vi "溶解氧电极校准.vi"() -> ()   [LabVIEW 2016, in "斯坦道多参数.lvlib"]
uses:
  <vilib>/Utility/miscctls.llb/LVPointTypeDef.ctl
  <vilib>/Analysis/NI_AALBase.lvlib
panel:
  out "第二点校准值":dbl
  out "第一点校准值":dbl
  out "最小值":sgl format="%#.2f"
  out "最大值":sgl format="%#.2f"
  in  "校准模式":enum16{"两点校准", "单点校准"}(ring)=enum."单点校准"
  in  "校准停止":bool
  in  "校准启动":bool
  out "波形图表":sgl(graph) caption="历史曲线"
  out "变异系数":dbl format="%#.6f"
  out "standard deviation":dbl caption="标准差" format="%#.2f"
  out "mean":dbl caption="均值" format="%#.2f"
  out "测量读值":dbl
  out "偏移值补偿":dbl
  out "饱和度值":dbl
  out "提示":string
  out "气压补偿值":dbl
  out "盐度补偿值":dbl
  out "电极斜率":dbl
  out "电极零点":dbl
  # "溶解氧电极设定"
  # "%"
  # "%"
  # "%"
  # "mg/L"
  # "ppt"
  # "hPa"
  # "mg/L"
  # "请选择校准模式:"
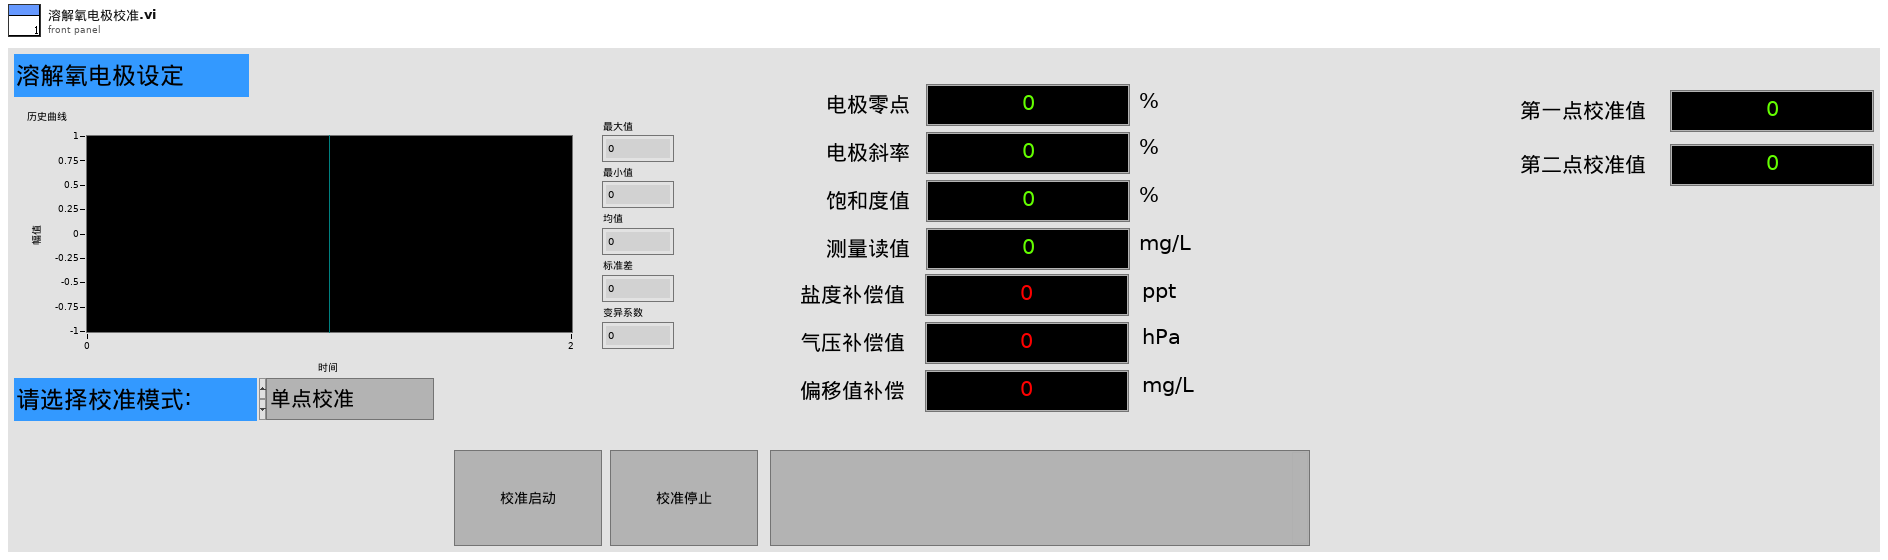
[diagram p1: front panel]
types:
  T1 = typedef "斯坦道多参数.lvlib/校准步骤.ctl" = enum16{"待机", "放置第一点标液", "第一点校准启动", "第一点校准写入", "第一点校准失败", "放置第二点标液", "第二点校准启动", "第二点校准写入", "第二点校准失败", "校准结果写入", "校准结束"}
  T2 = typedef "LVPointTypeDef.ctl" = cluster{"Horizontal":i16, "Vertical":i16}
  T3 = cluster{"电极状态标志":u16, "电极型号标志":u16, "溶解氧测量值":sgl, "温度测量值":sgl, "溶解氧饱和度值":sgl, "盐度补偿值":sgl, "大气压补偿值":sgl, "溶解氧偏移修正值":sgl, "温度偏移修正值":sgl, "手动温度补偿值":sgl, "溶解氧电极零点":sgl, "溶解氧电极斜率":sgl, "第1点标准值记录":sgl, "第1点信号值记录":sgl, "第1点温度值记录":sgl, "第2点标准值记录":sgl, "第2点信号值记录":sgl, "第2点温度值记录":sgl, "命令滤波设定":u16, "温度模式":enum16{"ATC", "MTC"}, "生产批次":u16, "电极序号":u16, "串口地址":u16, "串口波特率":enum16{"9600", "19200", "115200"}, "串口校验位":enum16{"NONE", "ODD", "EVEN"}, "串口停止位":enum16{"1bit", "2bit"}, "第一点标准值":sgl, "第二点标准值":sgl}
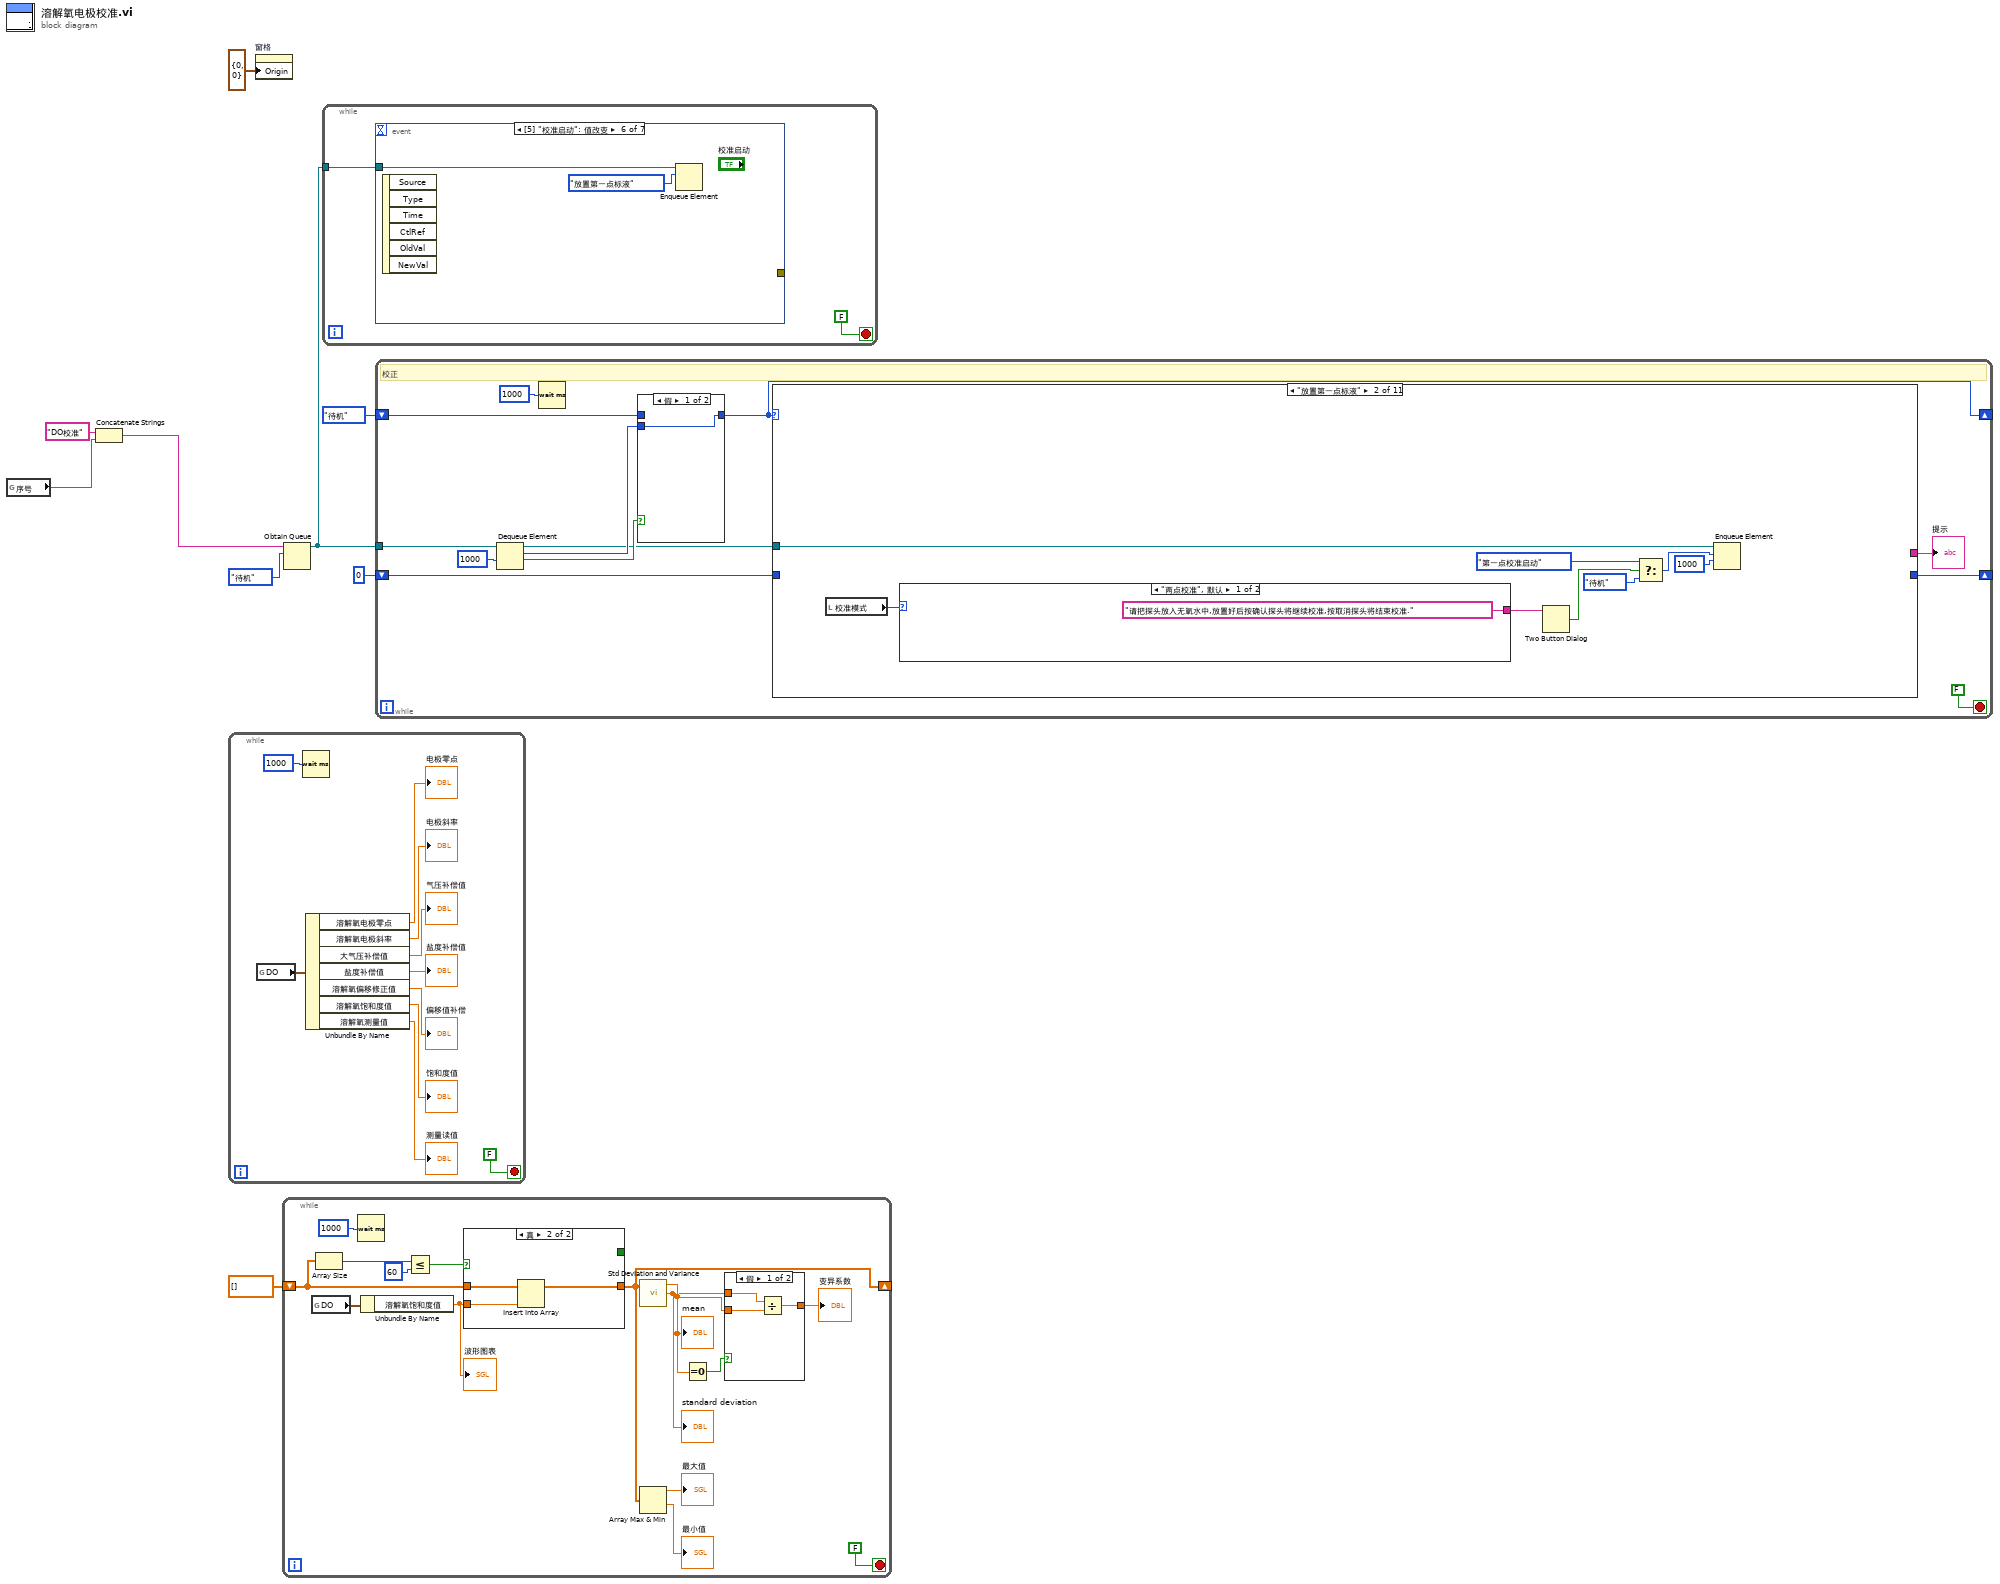
[diagram p0: block diagram]
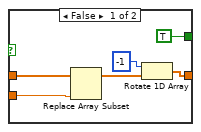
[diagram p3: hidden frame]
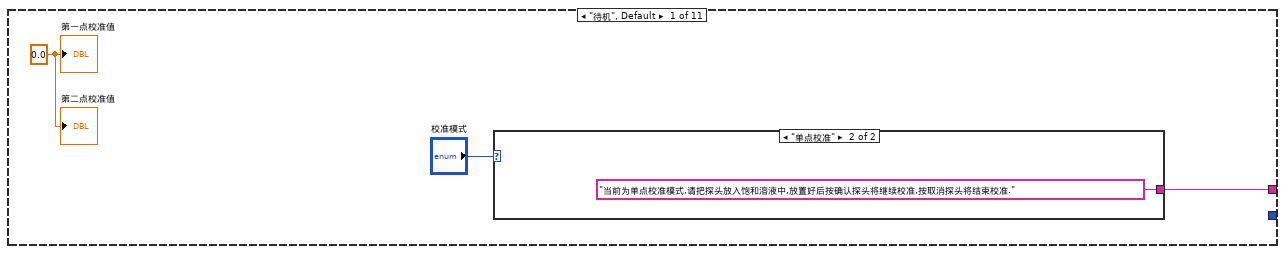
[diagram p5: hidden frame]
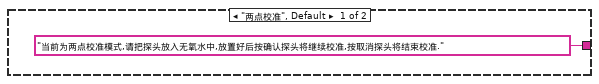
[diagram p6: hidden frame]
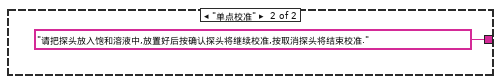
[diagram p7: hidden frame]
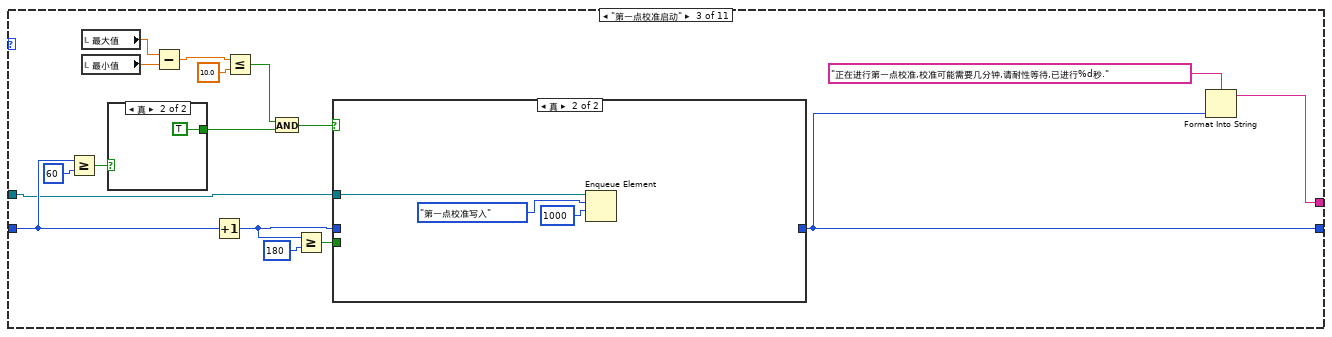
[diagram p8: hidden frame]
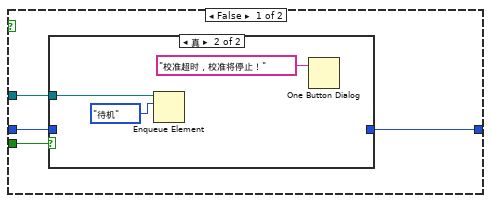
[diagram p9: hidden frame]
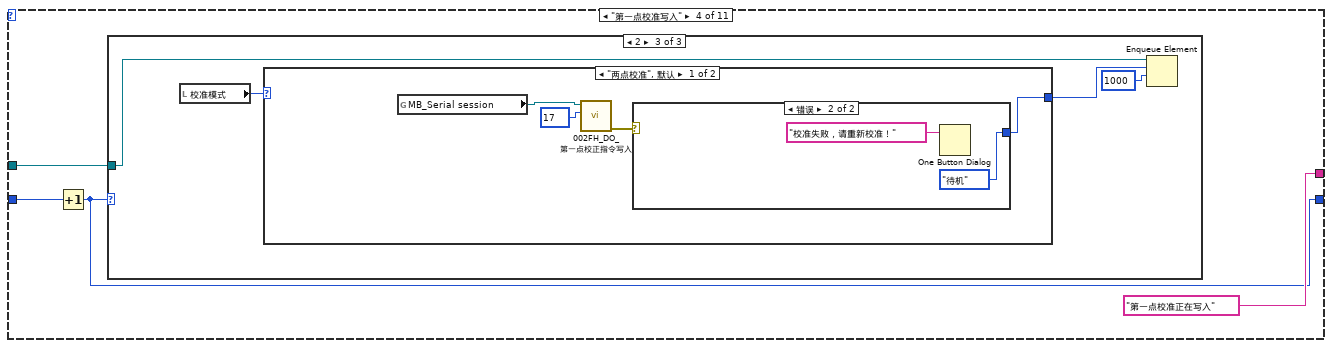
[diagram p12: hidden frame]
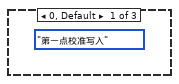
[diagram p13: hidden frame]
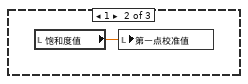
[diagram p14: hidden frame]
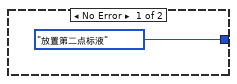
[diagram p15: hidden frame]
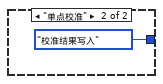
[diagram p16: hidden frame]
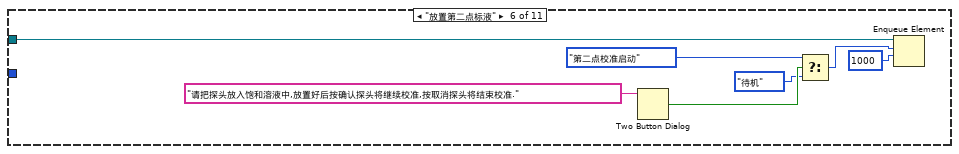
[diagram p18: hidden frame]
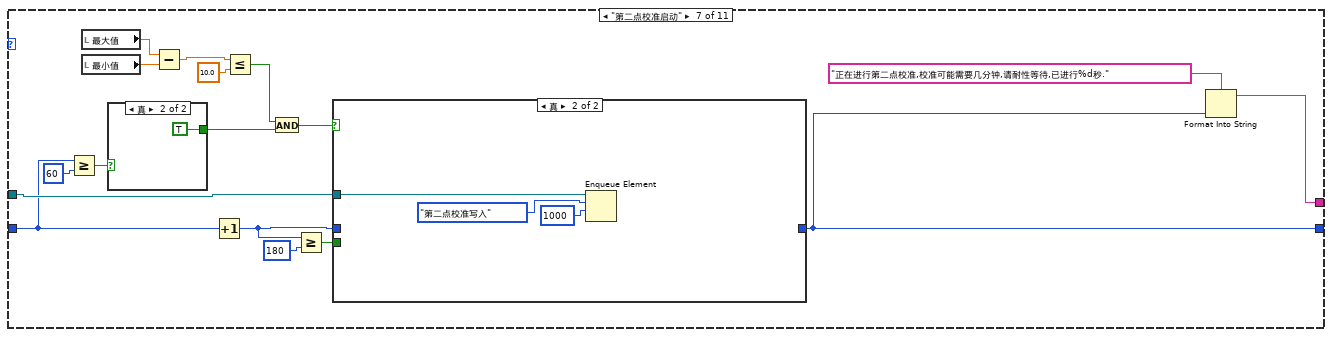
[diagram p19: hidden frame]
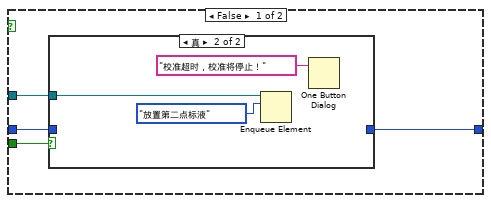
[diagram p20: hidden frame]
diagram:
  n1 = global read "多参数全局变量.vi" "序号"() -> (w1:string)
  n2 = Concatenate Strings("DO校准" ("名称（未命名）"), w1) -> (w2:string)
  n3 = while {
    stop <- FALSE stop-if-true
    n4 = global read "国弘过程全局变量.vi" "DO"() -> (w17:T3)
    n5 = Wait (ms)(milliseconds to wait=u32 1000 ("等待时间（毫秒）")) -> ()  [unwired: 1 out]
    n6 = Unbundle By Name(w17) -> ("溶解氧电极零点"=→"电极零点":sgl, "溶解氧电极斜率"=→"电极斜率":sgl, "大气压补偿值"=→"气压补偿值":sgl, "盐度补偿值"=→"盐度补偿值":sgl, "溶解氧偏移修正值"=→"偏移值补偿":sgl, "溶解氧饱和度值"=→"饱和度值":sgl, "溶解氧测量值"=→"测量读值":sgl)
  }
  n7 = property on="窗格" class="Pane"("Origin"=T2 {"Horizontal"=0, "Vertical"=0} ("原点")) -> ()  [unwired: 2 in, 2 out]
  n8 = while {
    shift-right: [w23] -> _
    shift-left: sgl[] [] -> [w30]
    stop <- FALSE stop-if-true
    n9 = global read "国弘过程全局变量.vi" "DO"() -> (w26:T3)
    n10 = Array Size(array=w30) -> (size(s)=w32:i32)
    n11 = Wait (ms)(milliseconds to wait=u32 1000 ("等待时间（毫秒）")) -> ()  [unwired: 1 out]
    n12 = Unbundle By Name(w26) -> ("溶解氧饱和度值"=w20:sgl)
    "波形图表" <- w20
    n13 = Less Or Equal?(x=w32, y=60) -> (x <= y?=w31:bool)
    n14 = case shown="真" w31 {
      tunnel: w30 -> [w43 w46]
      tunnel: w20 -> [w41 w45]
      tunnel: [w39 w44] -> w23
      tunnel: [TRUE _] -> _
      frame False {
        n15 = Replace Array Subset(array=w43, new element=w41) -> (w42:sgl[])  [unwired: 1 in]
        n16 = Rotate 1D Array(1:w42, 2:-1 ("n")) -> (0:w39:sgl[])
      }
      frame True {
        n17 = Insert Into Array(array=w46, new element=w45) -> (w44:sgl[])  [unwired: 1 in]
      }
    }
    n18 = call <vilib>:"Std Deviation and Variance.vi"("X"=w23) -> ("mean"=w25:dbl, "standard deviation"=w24:dbl)  [unwired: 1 in, 1 out]
    "mean" <- w25
    "standard deviation" <- w24
    n19 = Array Max & Min(array=w23) -> (max value=→"最大值":sgl, min value=→"最小值":sgl)  [unwired: 2 out]
    n20 = Equal To 0?(x=w25) -> (x = 0?=w29:bool)
    n21 = case shown="假" w29 {
      tunnel: w24 -> [w37 _]
      tunnel: [w36 _] -> w28
      tunnel: w25 -> [w35 _]
      frame False {
        n22 = Divide(x=w37, y=w35) -> (x/y=w36:dbl)
      }
      frame True {
      }
    }
    "变异系数" <- w28
  }
  n23 = Obtain Queue(name (unnamed)=w2, element data type=校准步骤."待机" ("枚举")) -> (queue out=w3:refnum<queue>)  [unwired: 3 in, 2 out]
  n24 = while {
    tunnel: w3 -> [w47]
    stop <- FALSE stop-if-true
    n25 = event shown="[5] \"校准启动\": 值改变" {
      selector: _ -> [_ _ _ _ _ _ _]
      dyn-events: _ -> [_ _ _ _ _ _ _]
      timeout: _ -> [_ _ _ _ _ _ _]
      tunnel: [_ _ w54 w57 w60 _ _] -> _
      tunnel: w47 -> [_ _ _ _ _ w62 w64]
      event Timeout {
        n26 = event-data() -> ()  [unwired: 1 in, 3 out]
      }
      event "盐度补偿值", "气压补偿值", "偏移值补偿": Mouse Down {
        n27 = event-data() -> ("CtlRef"=w50:refnum<vi>)  [unwired: 1 in, 7 out]
        n28 = property class="DigNum (严格)"(reference=w50) -> (reference out=w49:refnum<vi>, "Value"=w51:dbl)  [unwired: 1 in, 1 out]
        n29 = call "数字键盘.vi"("OldNumber"=w51) -> ("NewNumber"=w52:sgl)
        n30 = property class="DigNum (严格)"(reference=w49, "Val(Sgnl)"=w52) -> ()  [unwired: 1 in, 2 out]
      }
      event "盐度补偿值": Value Change {
        n31 = event-data() -> ("NewVal"=w55:dbl)  [unwired: 1 in, 5 out]
        n32 = global read "多参数全局变量.vi" "MB_Serial session"() -> (w53:refnum<class "MB_Master_Serial.lvclass">)
        n33 = call "0008H_DO_盐度补偿值写入.vi"("数值"=w55, "MB_Serial session in"=w53) -> ("error out"=w54:errorcluster)  [unwired: 8 in, 1 out]
      }
      event "气压补偿值": Value Change {
        n34 = event-data() -> ("NewVal"=w58:dbl)  [unwired: 1 in, 5 out]
        n35 = global read "多参数全局变量.vi" "MB_Serial session"() -> (w56:refnum<class "MB_Master_Serial.lvclass">)
        n36 = call "000AH_DO_大气压补偿值写入.vi"("数值"=w58, "MB_Serial session in"=w56) -> ("error out"=w57:errorcluster)  [unwired: 8 in, 1 out]
      }
      event "偏移值补偿": Value Change {
        n37 = event-data() -> ("NewVal"=w61:dbl)  [unwired: 1 in, 5 out]
        n38 = global read "多参数全局变量.vi" "MB_Serial session"() -> (w59:refnum<class "MB_Master_Serial.lvclass">)
        n39 = call "000CH_DO_DO偏移修正值写入.vi"("数值"=w61, "MB_Serial session in"=w59) -> ("error out"=w60:errorcluster)  [unwired: 8 in, 1 out]
      }
      event "校准启动": Value Change {
        n40 = event-data() -> ()  [unwired: 1 in, 6 out]
        n41 = Enqueue Element(queue=w62, element=校准步骤."放置第一点标液" ("元素")) -> ()  [unwired: 2 in, 3 out]
      }
      event "校准停止": Value Change {
        n42 = event-data() -> ()  [unwired: 1 in, 6 out]
        n43 = Flush Queue(queue=w64) -> (queue out=w65:refnum<queue>)  [unwired: 1 in, 2 out]
        n44 = Enqueue Element(queue=w65, element=校准步骤."待机" ("元素"), timeout in ms (-1)=1000 ("超时毫秒(-1)")) -> ()  [unwired: 1 in, 3 out]
      }
    }
  }
  n45 = while "While循环" {
    shift-right: [w69] -> _
    shift-left: 校准步骤."待机" ("枚举") -> [w70]
    shift-right: [w76] -> _
    shift-left: 0 -> [w77]
    tunnel: w3 -> [w71]
    stop <- FALSE stop-if-true
    # "校正"
    n46 = Dequeue Element(queue=w71, timeout in ms (-1)=1000 ("超时毫秒(-1)")) -> (queue out=w68:refnum<queue>, element=w72:T1, timed out?=w73:bool)  [unwired: 1 in, 1 out]
    n47 = Wait (ms)(milliseconds to wait=u32 1000 ("等待时间（毫秒）")) -> ()  [unwired: 1 out]
    n48 = case shown="假" w73 {
      tunnel: w72 -> [w80 _]
      tunnel: [w80 w81] -> w69
      tunnel: w70 -> [_ w81]
      frame False {
      }
      frame True {
      }
    }
    n49 = case shown="\"放置第一点标液\"" w69 {
      tunnel: [w84 _ w101 "第一点校准正在写入" ("提示") _ _ w151 "第二点校准正在写入" ("提示") _ w193 w221] -> w75
      tunnel: w77 -> [_ _ w105 w128 _ _ w153 w181 _ _ _]
      tunnel: [_ _ w104 w127 _ _ w152 w180 _ _ _] -> w76
      tunnel: w68 -> [_ w88 w103 w126 _ w143 w154 w179 _ w195 _]
      frame "待机", Default {
        w82 = 0.0 ("第一点校准值")
        n50 = case shown="\"单点校准\"" "校准模式" {
          tunnel: ["当前为两点校准模式,请把探头放入无氧水中,放置好后按确认探头将继续校准,按取消探头将结束校准." ("消息") "当前为单点校准模式,请把探头放入饱和溶液中,放置好后按确认探头将继续校准,按取消探头将结束校准." ("消息")] -> w84
          frame "两点校准", Default {
          }
          frame "单点校准" {
          }
        }
        "第一点校准值" <- w82
        "第二点校准值" <- w82
      }
      frame "放置第一点标液" {
        n51 = local read "校准模式"() -> (w87:enum16{"两点校准", "单点校准"})
        n52 = case shown="\"两点校准\", 默认" w87 {
          tunnel: ["请把探头放入无氧水中,放置好后按确认探头将继续校准,按取消探头将结束校准." ("消息") "请把探头放入饱和溶液中,放置好后按确认探头将继续校准,按取消探头将结束校准." ("消息")] -> w94
          frame "两点校准", Default {
          }
          frame "单点校准" {
          }
        }
        n53 = Two Button Dialog(message=w94) -> (T button?=w92:bool)  [unwired: 2 in]
        n54 = Select(t=校准步骤."第一点校准启动" ("元素"), s=w92, f=校准步骤."待机" ("元素")) -> (s? t:f=w89:T1)
        n55 = Enqueue Element(queue=w88, element=w89, timeout in ms (-1)=1000 ("超时毫秒(-1)")) -> ()  [unwired: 1 in, 3 out]
      }
      frame "第一点校准启动" {
        n56 = Greater Or Equal?(x=w105, y=60) -> (x >= y?=w112:bool)
        n57 = local read "最大值"() -> (w109:sgl)
        n58 = local read "最小值"() -> (w108:sgl)
        n59 = case shown="真" w112 {
          tunnel: [_ TRUE] -> w100
          frame False {
          }
          frame True {
          }
        }
        n60 = Subtract(x=w109, y=w108) -> (x-y=w110:sgl)
        n61 = Increment(x=w105) -> (x+1=w102:i32)
        n62 = Less Or Equal?(x=w110, y=10.0) -> (x <= y?=w99:bool)
        n63 = And(x=w99, y=w100) -> (x .and. y?=w98:bool)
        n64 = Greater Or Equal?(x=w102, y=180) -> (x >= y?=w106:bool)
        n65 = case shown="真" w98 {
          tunnel: w103 -> [w116 w124]
          tunnel: w106 -> [w117 _]
          tunnel: w102 -> [w115 _]
          tunnel: [w114 _] -> w104
          frame False {
            n66 = case shown="真" w117 {
              tunnel: w116 -> [_ w121]
              tunnel: w115 -> [w118 _]
              tunnel: [w118 _] -> w114
              frame False {
              }
              frame True {
                n67 = Enqueue Element(queue=w121, element=校准步骤."待机" ("元素")) -> ()  [unwired: 2 in, 3 out]
                n68 = One Button Dialog(message="校准超时，校准将停止！" ("消息")) -> ()  [unwired: 1 in, 1 out]
              }
            }
          }
          frame True {
            n69 = Enqueue Element(queue=w124, element=校准步骤."第一点校准写入" ("元素"), timeout in ms (-1)=1000 ("超时毫秒(-1)")) -> ()  [unwired: 1 in, 3 out]
          }
        }
        n70 = Format Into String(format string="正在进行第一点校准,校准可能需要几分钟,请耐性等待,已进行%d秒." ("格式字符串"), w104) -> (resulting string=w101:string)  [unwired: 2 in, 1 out]
      }
      frame "第一点校准写入" {
        n71 = Increment(x=w128) -> (x+1=w127:i32)
        n72 = case shown="2" w127 {
          tunnel: w126 -> [_ _ w132]
          frame 0, Default {
            (unwired) 校准步骤."第一点校准写入" ("枚举")
          }
          frame 1 {
            n73 = local read "饱和度值"() -> (w130:dbl)
            n74 = local write "第一点校准值"(w130) -> ()
          }
          frame 2 {
            n75 = local read "校准模式"() -> (w134:enum16{"两点校准", "单点校准"})
            n76 = case shown="\"两点校准\", 默认" w134 {
              tunnel: [w135 校准步骤."校准结果写入" ("枚举")] -> w131
              frame "两点校准", Default {
                n77 = global read "多参数全局变量.vi" "MB_Serial session"() -> (w136:refnum<class "MB_Master_Serial.lvclass">)
                n78 = call "002FH_DO_第一点校正指令写入.vi"("数值"=u16 17, "MB_Serial session in"=w136) -> ("error out"=w137:errorcluster)  [unwired: 8 in, 1 out]
                n79 = case shown="错误" w137 {
                  tunnel: [校准步骤."放置第二点标液" ("元素") 校准步骤."待机" ("元素")] -> w135
                  frame No Error {
                  }
                  frame Error {
                    n80 = One Button Dialog(message="校准失败，请重新校准！" ("消息")) -> ()  [unwired: 1 in, 1 out]
                  }
                }
              }
              frame "单点校准" {
              }
            }
            n81 = Enqueue Element(queue=w132, element=w131, timeout in ms (-1)=1000 ("超时毫秒(-1)")) -> ()  [unwired: 1 in, 3 out]
          }
        }
      }
      frame "第一点校准失败" {
      }
      frame "放置第二点标液" {
        n82 = Two Button Dialog(message="请把探头放入饱和溶液中,放置好后按确认探头将继续校准,按取消探头将结束校准." ("消息")) -> (T button?=w147:bool)  [unwired: 2 in]
        n83 = Select(t=校准步骤."第二点校准启动" ("元素"), s=w147, f=校准步骤."待机" ("元素")) -> (s? t:f=w144:T1)
        n84 = Enqueue Element(queue=w143, element=w144, timeout in ms (-1)=1000 ("超时毫秒(-1)")) -> ()  [unwired: 1 in, 3 out]
      }
      frame "第二点校准启动" {
        n85 = Greater Or Equal?(x=w153, y=60) -> (x >= y?=w165:bool)
        n86 = local read "最大值"() -> (w162:sgl)
        n87 = local read "最小值"() -> (w161:sgl)
        n88 = case shown="真" w165 {
          tunnel: [_ TRUE] -> w158
          frame False {
          }
          frame True {
          }
        }
        n89 = Subtract(x=w162, y=w161) -> (x-y=w163:sgl)
        n90 = Increment(x=w153) -> (x+1=w159:i32)
        n91 = Less Or Equal?(x=w163, y=10.0) -> (x <= y?=w157:bool)
        n92 = And(x=w157, y=w158) -> (x .and. y?=w156:bool)
        n93 = Greater Or Equal?(x=w159, y=180) -> (x >= y?=w160:bool)
        n94 = case shown="真" w156 {
          tunnel: w154 -> [w169 w177]
          tunnel: w160 -> [w170 _]
          tunnel: w159 -> [w168 _]
          tunnel: [w167 _] -> w152
          frame False {
            n95 = case shown="真" w170 {
              tunnel: w169 -> [_ w174]
              tunnel: w168 -> [w171 _]
              tunnel: [w171 _] -> w167
              frame False {
              }
              frame True {
                n96 = Enqueue Element(queue=w174, element=校准步骤."放置第二点标液" ("元素")) -> ()  [unwired: 2 in, 3 out]
                n97 = One Button Dialog(message="校准超时，校准将停止！" ("消息")) -> ()  [unwired: 1 in, 1 out]
              }
            }
          }
          frame True {
            n98 = Enqueue Element(queue=w177, element=校准步骤."第二点校准写入" ("元素"), timeout in ms (-1)=1000 ("超时毫秒(-1)")) -> ()  [unwired: 1 in, 3 out]
          }
        }
        n99 = Format Into String(format string="正在进行第二点校准,校准可能需要几分钟,请耐性等待,已进行%d秒." ("格式字符串"), w152) -> (resulting string=w151:string)  [unwired: 2 in, 1 out]
      }
      frame "第二点校准写入" {
        n100 = Increment(x=w181) -> (x+1=w180:i32)
        n101 = case shown="2" w180 {
          tunnel: w179 -> [_ _ w184]
          frame 0, Default {
            (unwired) 校准步骤."第二点校准写入" ("枚举")
          }
          frame 1 {
            n102 = local read "饱和度值"() -> (w183:dbl)
            n103 = local write "第二点校准值"(w183) -> ()
          }
          frame 2 {
            n104 = global read "多参数全局变量.vi" "MB_Serial session"() -> (w188:refnum<class "MB_Master_Serial.lvclass">)
            n105 = call "0032H_DO_第二点校正指令写入.vi"("数值"=u16 33, "MB_Serial session in"=w188) -> ("error out"=w185:errorcluster)  [unwired: 8 in, 1 out]
            n106 = case shown="无错误" w185 {
              tunnel: [校准步骤."校准结果写入" ("元素") 校准步骤."放置第二点标液" ("元素")] -> w186
              frame No Error {
              }
              frame Error {
                n107 = One Button Dialog(message="校准失败，请重新校准！" ("消息")) -> ()  [unwired: 1 in, 1 out]
              }
            }
            n108 = Enqueue Element(queue=w184, element=w186, timeout in ms (-1)=1000 ("超时毫秒(-1)")) -> ()  [unwired: 1 in, 3 out]
          }
        }
      }
      frame "第二点校准失败" {
      }
      frame "校准结果写入" {
        n109 = Enqueue Element(queue=w195, element=校准步骤."校准结束" ("元素")) -> ()  [unwired: 2 in, 3 out]
        n110 = local read "校准模式"() -> (w194:enum16{"两点校准", "单点校准"})
        n111 = case shown="\"两点校准\", 默认" w194 {
          tunnel: [w197 w213] -> w193
          frame "两点校准", Default {
            n112 = global read "国弘过程全局变量.vi" "DO"() -> (w199:T3)
            n113 = Unbundle By Name(w199) -> ("电极状态标志"=w198:u16)
            n114 = case shown="2" w198 {
              selector: w198 -> [w201 _ w210]
              tunnel: [w200 w205 w209] -> w197
              frame 0, Default {
                n115 = case shown="1" w201 {
                  tunnel: ["校正未正常启动，请重新校正" "第一点校准通过" "第二点校准通过"] -> w200
                  frame 0, Default {
                  }
                  frame 1 {
                  }
                  frame 2 {
                  }
                }
              }
              frame 2 {
                n116 = local read "第一点校准值"() -> (w207:dbl)
                n117 = local read "第二点校准值"() -> (w208:dbl)
                n118 = Format Into String(format string="两点校准结果：\n第一点校准值：%f\n第二点校准值：%f" ("提示"), w207, w208) -> (resulting string=w205:string)  [unwired: 2 in, 1 out]
              }
              frame 3, 4 {
                n119 = case shown="4" w210 {
                  tunnel: ["校正失败，电极零点超出范围" "校正失败，电极斜率超出范围"] -> w209
                  frame 3, Default {
                  }
                  frame 4 {
                  }
                }
              }
            }
          }
          frame "单点校准" {
            n120 = global read "多参数全局变量.vi" "MB_Serial session"() -> (w215:refnum<class "MB_Master_Serial.lvclass">)
            n121 = call "0032H_DO_第二点校正指令写入.vi"("数值"=u16 33, "MB_Serial session in"=w215) -> ("error out"=w214:errorcluster)  [unwired: 8 in, 1 out]
            n122 = case shown="无错误" w214 {
              tunnel: [w217 "校准失败，请重新校准！" ("消息")] -> w213
              frame No Error {
                n123 = local read "第一点校准值"() -> (w218:dbl)
                n124 = Format Into String(format string="单点校准结果：\n校准值：%f" ("提示"), w218) -> (resulting string=w217:string)  [unwired: 2 in, 1 out]
              }
              frame Error {
              }
            }
          }
        }
        n125 = One Button Dialog(message=w193) -> ()  [unwired: 1 in, 1 out]
      }
      frame "校准结束" {
        n126 = local read "提示"() -> (w221:string)
      }
    }
    "提示" <- w75
  }
